vi "Init.vi"(8 "error in (no error)":errorcluster, 11 "Data in":refnum<class "Blackboard_String.lvclass">) -> (0 "error out":errorcluster, 3 "Data out":refnum<class "Blackboard_String.lvclass">)   [LabVIEW 2021, in "Blackboard_String.lvclass"]
doc: "Abstract Data Classes 2.1.1.12\nTim Streeter - TSA\nCopyright (c) 2024, TSA"
uses:
  Blackboard_String.lvclass
  C:/Program Files (x86)/National Instruments/LabVIEW 2021/vi.lib/TSA/Abstract Data Classes/Abs_Types/Type/Abs_Type.lvclass
  Blackboard_String.lvclass/Blackboard_String.ctl
  <vilib>/TSA/Abstract Data Classes/Abs_Types/Type/Abs_Type.lvclass/Abs_Type.ctl
  Data Type.ctl
  Blackboard.lvclass/Blackboard.ctl
  Properties/Read Blackboard.vi
  Properties/Read Group.vi
  Properties/Read Write.vi
  Properties/Write Blackboard.vi
  Properties/Write Tag Index.vi
  Properties/Write Group Index.vi
  Initialise DVRs.vi
  <vilib>/Utility/error.llb/Error Cluster From Error Code.vi
  Blackboard.lvclass
  <vilib>/TSA/Abstract Data Classes/Abs_Types/Type/Abs_Type.lvclass
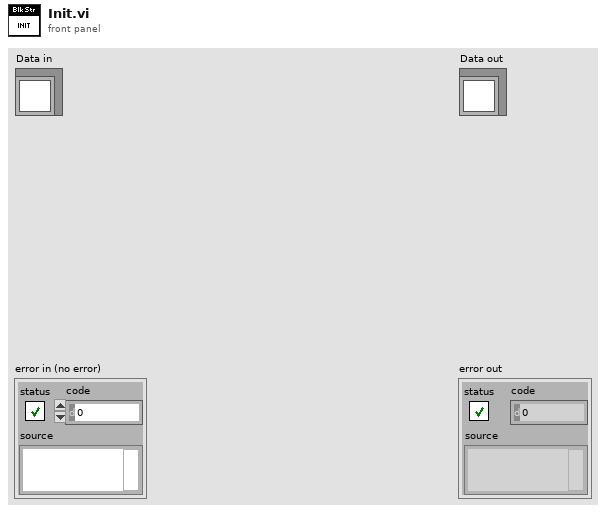
[diagram p1: front panel]
types:
  T1 = typedef "Blackboard.lvclass/Data Type.ctl" = enum16{"Boolean", "String", "DBL", "SGL", "EXT", "U8", "U16", "U32", "U64", "I8", "I16", "I32", "I64", "CDBL", "CSGL", "CEXT", "Time", "Variant", "Waveform"}
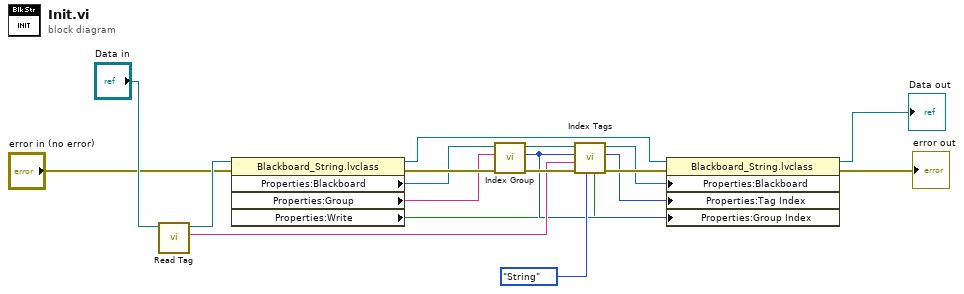
[diagram p0: block diagram]
diagram:
  n1 = call <vilib>:"Read Tag.vi"("Abs_Type in"="Data in") -> ("Tag"=w13:string, "Abs_Type out"=w15:refnum<class "Blackboard_String.lvclass">)  [unwired: 9 in]
  n2 = property class="Blackboard_String.lvclass"(reference=w15, error in="error in (no error)") -> (reference out=w2:refnum<class "Blackboard_String.lvclass">, error out=w17:errorcluster, "Properties:Blackboard"=w11:refnum<class "Blackboard.lvclass">, "Properties:Group"=w10:string, "Properties:Write"=w1:bool)
  n3 = call "Index Group.vi"("error in (no error)"=w17, "Group"=w10, "bt_Blackboard in"=w11) -> ("error out"=w16:errorcluster, "Index"=w5:i32, "bt_Blackboard out"=w18:refnum<class "Blackboard.lvclass">)  [unwired: 6 in]
  n4 = call "Index Tags.vi"("Write?"=w1, "Data Type"=Data_Type."String", "error in (no error)"=w16, "Tag"=w13, "Group Index"=w5, "bt_Blackboard in"=w18) -> ("error out"=w8:errorcluster, "Index"=w6:i32, "bt_Blackboard out"=w7:refnum<class "Blackboard.lvclass">)  [unwired: 2 in, 1 out]
  n5 = property class="Blackboard_String.lvclass"(reference=w2, error in=w8, "Properties:Blackboard"=w7, "Properties:Tag Index"=w6, "Properties:Group Index"=w5) -> (reference out=→"Data out":refnum<class "Blackboard_String.lvclass">, error out=→"error out":errorcluster)
